vi "LM3Sxxxx_PWM_Config.vi"(8 "error in (no error)":errorcluster, 10 "Config Data":string[](array[string]), 11 "Interrupt Name":string) -> (0 "error out":errorcluster, 3 "Interrupt Configuration":string[](array[string]))   [LabVIEW 2011]
panel:
  in  "PWM 1":string
  in  "PWM 0":string
  in  "Invert output":bool
  in  "Disable on fault":bool
  in  "Invert output":bool
  in  "Disable on fault":bool
  in  "help":bool
  in  "Duty cycle units":u32(ring) items=["Percent", "Hundredths percent", "PWM duty cycle"]
  in  "Duty cycle units":u32(ring) items=["Percent", "Hundredths percent", "PWM duty cycle"]
  in  "Duty cycle":u32=50
  in  "Duty cycle":u32=50
  in  "Enable":bool
  in  "Enable":bool=TRUE
  in  "Zero":bool
  in  "Compare B":bool
  in  "Compare A":bool
  in  "Load":bool
  in  "Center alignment":bool
  in  "Frequency (Hz)":u32=1000
  in  "cancel":bool
  in  "ok":bool
  in  "PWM divider":u32(ring) items=["/1", "/2", "/4", "/8", "/16", "/32", "/64"]
  # "Interrupts"
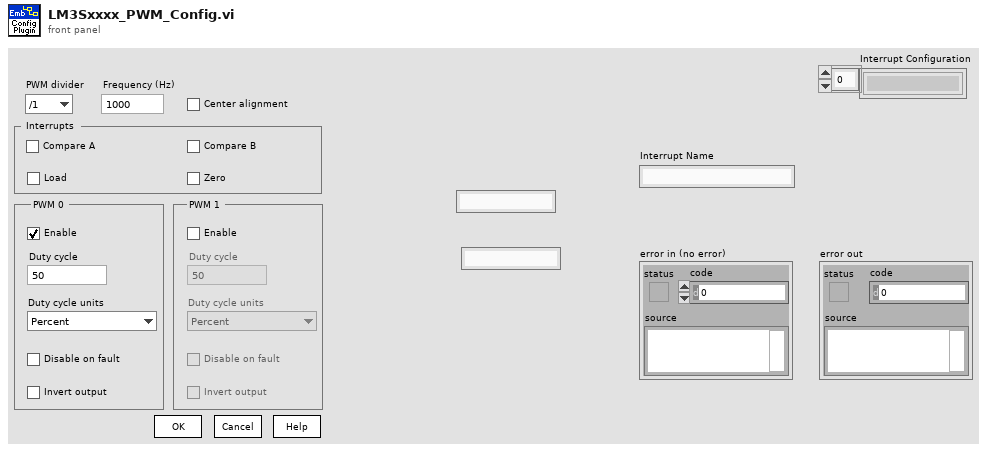
[diagram p1: front panel]
types:
  T1 = enum8{"Enabled", "Disabled", "Disabled and Grayed Out"}
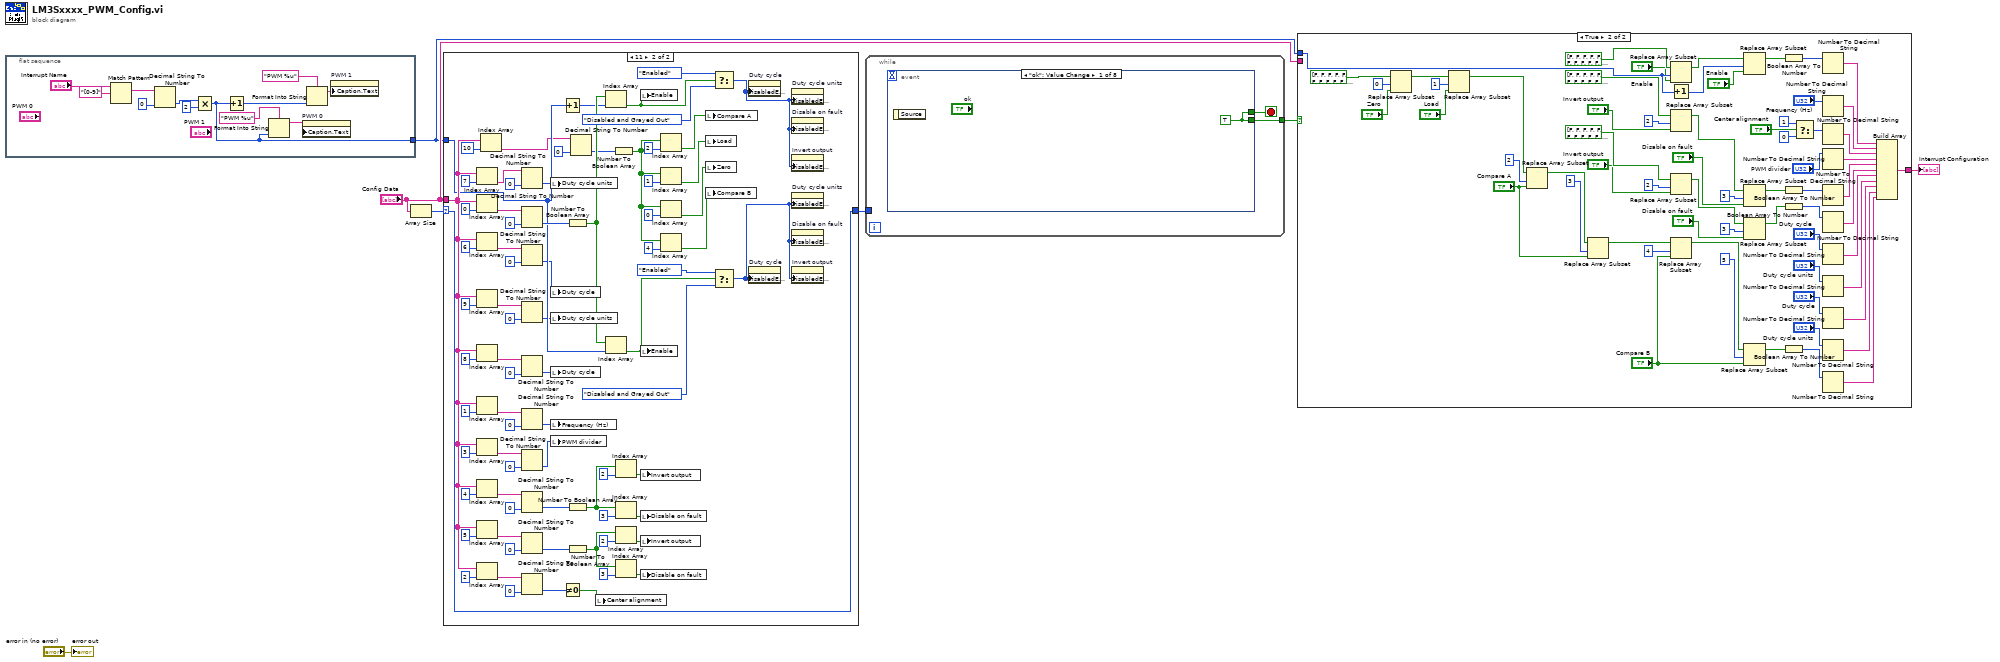
[diagram p0: block diagram]
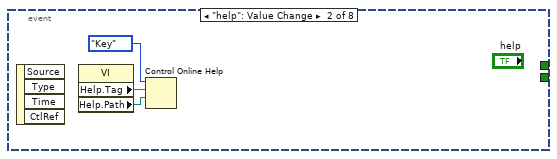
[diagram p4: hidden frame]
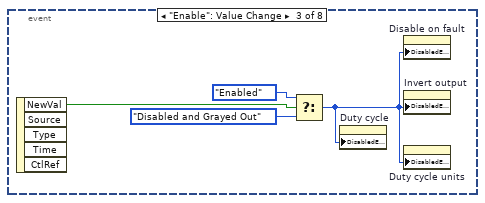
[diagram p5: hidden frame]
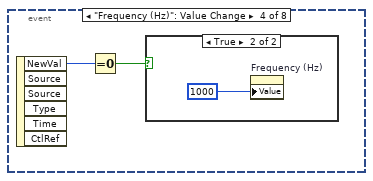
[diagram p6: hidden frame]
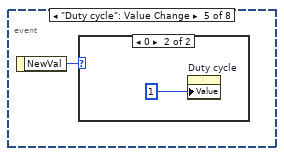
[diagram p8: hidden frame]
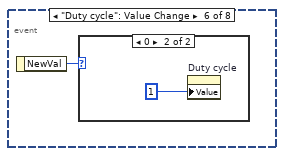
[diagram p10: hidden frame]
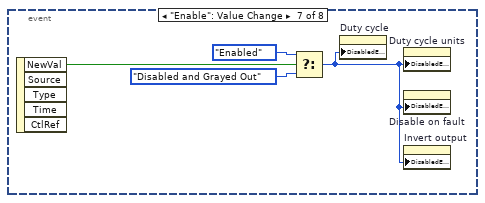
[diagram p12: hidden frame]
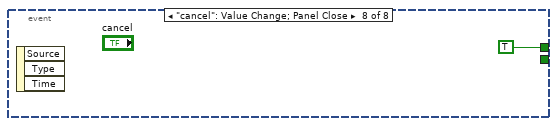
[diagram p13: hidden frame]
diagram:
  n1 = flat-sequence {
    tunnel: [w10] -> w1
    frame #0 {
      n2 = Match Pattern(string="Interrupt Name", regular expression="[0-9]") -> (match substring=w16:string)  [unwired: 1 in, 3 out]
      n3 = Decimal String To Number(string=w16, default (0L)=u32 0) -> (number=w9:u32)  [unwired: 1 in, 1 out]
      n4 = Multiply(x=w9, y=2) -> (x*y=w10:u32)
      n5 = Increment(x=w10) -> (x+1=w12:u32)
      n6 = Format Into String(format string="PWM %u", w10) -> (resulting string=w14:string)  [unwired: 2 in, 1 out]
      n7 = property on="PWM 0" class="Str"("Caption.Text"=w14) -> ()  [unwired: 2 in, 2 out]
      n8 = Format Into String(format string="PWM %u", w12) -> (resulting string=w11:string)  [unwired: 2 in, 1 out]
      n9 = property on="PWM 1" class="Str"("Caption.Text"=w11) -> ()  [unwired: 2 in, 2 out]
    }
  }
  n10 = Array Size(array="Config Data") -> (size(s)=w4:i32)
  n11 = case shown="11" w4 {
    selector: w4 -> [w20 w85]
    tunnel: "Config Data" -> [_ w86]
    tunnel: [w20 w85] -> w2
    tunnel: w1 -> [_ w80]
    frame Default {
    }
    frame 11 {
      n12 = Index Array(array=w86, index=7) -> (element=w25:string)
      n13 = Index Array(array=w86, index=0) -> (element=w84:string)
      n14 = Index Array(array=w86, index=6) -> (element=w43:string)
      n15 = Index Array(array=w86, index=9) -> (element=w22:string)
      n16 = Index Array(array=w86, index=8) -> (element=w40:string)
      n17 = Index Array(array=w86, index=1) -> (element=w70:string)
      n18 = Index Array(array=w86, index=3) -> (element=w64:string)
      n19 = Index Array(array=w86, index=4) -> (element=w59:string)
      n20 = Index Array(array=w86, index=5) -> (element=w58:string)
      n21 = Index Array(array=w86, index=2) -> (element=w68:string)
      n22 = Index Array(array=w86, index=10) -> (element=w36:string)
      n23 = Decimal String To Number(string=w25, default (0L)=u32 0) -> (number=w24:u32)  [unwired: 1 in, 1 out]
      n24 = Decimal String To Number(string=w84, default (0L)=u32 0) -> (number=w83:u32)  [unwired: 1 in, 1 out]
      n25 = Decimal String To Number(string=w43, default (0L)=u32 0) -> (number=w42:u32)  [unwired: 1 in, 1 out]
      n26 = Decimal String To Number(string=w22, default (0L)=u32 0) -> (number=w21:u32)  [unwired: 1 in, 1 out]
      n27 = Decimal String To Number(string=w40, default (0L)=u32 0) -> (number=w39:u32)  [unwired: 1 in, 1 out]
      n28 = Decimal String To Number(string=w70, default (0L)=u32 0) -> (number=w69:u32)  [unwired: 1 in, 1 out]
      n29 = Decimal String To Number(string=w64, default (0L)=u32 0) -> (number=w63:u32)  [unwired: 1 in, 1 out]
      n30 = Decimal String To Number(string=w59, default (0L)=u32 0) -> (number=w57:u32)  [unwired: 1 in, 1 out]
      n31 = Decimal String To Number(string=w58, default (0L)=u32 0) -> (number=w56:u32)  [unwired: 1 in, 1 out]
      n32 = Decimal String To Number(string=w68, default (0L)=u32 0) -> (number=w66:u32)  [unwired: 1 in, 1 out]
      n33 = local write "Duty cycle units"(w24) -> ()
      n34 = local write "Duty cycle"(w42) -> ()
      n35 = local write "Duty cycle units"(w21) -> ()
      n36 = local write "Duty cycle"(w39) -> ()
      n37 = local write "Frequency (Hz)"(w69) -> ()
      n38 = local write "PWM divider"(w63) -> ()
      n39 = Increment(x=w80) -> (x+1=w79:u32)
      n40 = Not Equal To 0?(x=w66) -> (x != 0?=w65:bool)
      n41 = Number To Boolean Array(number=w83) -> (Boolean array=w81:bool[])
      n42 = Number To Boolean Array(number=w57) -> (Boolean array=w54:bool[])
      n43 = Number To Boolean Array(number=w56) -> (Boolean array=w53:bool[])
      n44 = Decimal String To Number(string=w36, default (0L)=u32 0) -> (number=w37:u32)  [unwired: 1 in, 1 out]
      n45 = local write "Center alignment"(w65) -> ()
      n46 = Index Array(array=w81, index=w79) -> (element=w72:bool)
      n47 = Index Array(array=w81, index=w80) -> (element=w76:bool)
      n48 = Number To Boolean Array(number=w37) -> (Boolean array=w35:bool[])
      n49 = Index Array(array=w54, index=2) -> (element=w48:bool)
      n50 = Index Array(array=w54, index=3) -> (element=w45:bool)
      n51 = Index Array(array=w53, index=2) -> (element=w47:bool)
      n52 = Index Array(array=w53, index=3) -> (element=w46:bool)
      n53 = local write "Enable"(w72) -> ()
      n54 = local write "Enable"(w76) -> ()
      n55 = local write "Invert output"(w48) -> ()
      n56 = local write "Disable on fault"(w45) -> ()
      n57 = local write "Invert output"(w47) -> ()
      n58 = local write "Disable on fault"(w46) -> ()
      n59 = Index Array(array=w35, index=2) -> (element=w32:bool)
      n60 = Index Array(array=w35, index=1) -> (element=w31:bool)
      n61 = Index Array(array=w35, index=0) -> (element=w34:bool)
      n62 = Index Array(array=w35, index=4) -> (element=w33:bool)
      n63 = local write "Compare A"(w32) -> ()
      n64 = local write "Load"(w31) -> ()
      n65 = local write "Zero"(w34) -> ()
      n66 = local write "Compare B"(w33) -> ()
      n67 = Select(t=T1."Enabled" ("Disabled"), s=w72, f=T1."Disabled and Grayed Out" ("Disabled")) -> (s? t:f=w75:T1)
      n68 = Select(t=T1."Enabled" ("Disabled"), s=w76, f=T1."Disabled and Grayed Out" ("Disabled")) -> (s? t:f=w78:T1)
      n69 = property on="Duty cycle" class="DigNum (strict)"("DisabledEnum"=w75) -> ()  [unwired: 2 in, 2 out]
      n70 = property on="Duty cycle" class="DigNum (strict)"("DisabledEnum"=w78) -> ()  [unwired: 2 in, 2 out]
      n71 = property on="Duty cycle units" class="Ring (strict)"("DisabledEnum"=w75) -> ()  [unwired: 2 in, 2 out]
      n72 = property on="Disable on fault" class="Bool (strict)"("DisabledEnum"=w75) -> ()  [unwired: 2 in, 2 out]
      n73 = property on="Invert output" class="Bool (strict)"("DisabledEnum"=w75) -> ()  [unwired: 2 in, 2 out]
      n74 = property on="Duty cycle units" class="Ring (strict)"("DisabledEnum"=w78) -> ()  [unwired: 2 in, 2 out]
      n75 = property on="Disable on fault" class="Bool (strict)"("DisabledEnum"=w78) -> ()  [unwired: 2 in, 2 out]
      n76 = property on="Invert output" class="Bool (strict)"("DisabledEnum"=w78) -> ()  [unwired: 2 in, 2 out]
    }
  }
  n77 = while {
    tunnel: [w98] -> w6
    tunnel: w2 -> [_]
    stop <- w99 stop-if-true
    n78 = event shown="[0] \"ok\": Value Change" {
      selector: _ -> [_ _ _ _ _ _ _ _]
      dyn-events: _ -> [_ _ _ _ _ _ _ _]
      timeout: _ -> [_ _ _ _ _ _ _ _]
      tunnel: [w100 _ _ _ _ _ _ TRUE] -> w99
      tunnel: [w100 _ _ _ _ _ _ _] -> w98
      event "ok": Value Change {
        w100 = TRUE
        n79 = event-data() -> ()  [unwired: 2 out]
      }
      event "help": Value Change {
        n80 = event-data() -> ()  [unwired: 5 out]
        n81 = property class="VI"() -> ("Help.Tag"=w101:string, "Help.Path"=w102:path)  [unwired: 2 in, 2 out]
        n82 = Control Online Help(2:w102, 3:w101, 4:enum16{"Contents", "Key", "Close"}."Key" ("Operation")) -> ()  [unwired: 1 in, 1 out]
      }
      event "Enable": Value Change {
        n83 = event-data() -> ("NewVal"=w104:bool)  [unwired: 5 out]
        n84 = Select(t=T1."Enabled" ("Disabled"), s=w104, f=T1."Disabled and Grayed Out" ("Disabled")) -> (s? t:f=w105:T1)
        n85 = property on="Duty cycle" class="DigNum (strict)"("DisabledEnum"=w105) -> ()  [unwired: 2 in, 2 out]
        n86 = property on="Disable on fault" class="Bool (strict)"("DisabledEnum"=w105) -> ()  [unwired: 2 in, 2 out]
        n87 = property on="Invert output" class="Bool (strict)"("DisabledEnum"=w105) -> ()  [unwired: 2 in, 2 out]
        n88 = property on="Duty cycle units" class="Ring (strict)"("DisabledEnum"=w105) -> ()  [unwired: 2 in, 2 out]
      }
      event "Frequency (Hz)": Value Change {
        n89 = event-data() -> ("NewVal"=w109:u32)  [unwired: 6 out]
        n90 = Equal To 0?(x=w109) -> (x = 0?=w108:bool)
        n91 = case shown="True" w108 {
          frame False {
          }
          frame True {
            n92 = property on="Frequency (Hz)" class="DigNum (strict)"("Value"=u32 1000 ("Frequency (Hz)")) -> ()  [unwired: 2 in, 2 out]
          }
        }
      }
      event "Duty cycle": Value Change {
        n93 = event-data() -> ("NewVal"=w111:u32)  [unwired: 1 out]
        n94 = case shown="0" w111 {
          frame Default {
          }
          frame 0 {
            n95 = property on="Duty cycle" class="DigNum (strict)"("Value"=u32 1 ("Duty cycle")) -> ()  [unwired: 2 in, 2 out]
          }
        }
      }
      event "Duty cycle": Value Change {
        n96 = event-data() -> ("NewVal"=w113:u32)  [unwired: 1 out]
        n97 = case shown="0" w113 {
          frame Default {
          }
          frame 0 {
            n98 = property on="Duty cycle" class="DigNum (strict)"("Value"=u32 1 ("Duty cycle")) -> ()  [unwired: 2 in, 2 out]
          }
        }
      }
      event "Enable": Value Change {
        n99 = event-data() -> ("NewVal"=w115:bool)  [unwired: 5 out]
        n100 = Select(t=T1."Enabled" ("Disabled"), s=w115, f=T1."Disabled and Grayed Out" ("Disabled")) -> (s? t:f=w116:T1)
        n101 = property on="Duty cycle" class="DigNum (strict)"("DisabledEnum"=w116) -> ()  [unwired: 2 in, 2 out]
        n102 = property on="Duty cycle units" class="Ring (strict)"("DisabledEnum"=w116) -> ()  [unwired: 2 in, 2 out]
        n103 = property on="Disable on fault" class="Bool (strict)"("DisabledEnum"=w116) -> ()  [unwired: 2 in, 2 out]
        n104 = property on="Invert output" class="Bool (strict)"("DisabledEnum"=w116) -> ()  [unwired: 2 in, 2 out]
      }
      event "cancel": Value Change; Panel Close {
        n105 = event-data() -> ()  [unwired: 4 out]
      }
    }
  }
  n106 = case shown="True" w6 {
    tunnel: "Config Data" -> [w120 _]
    tunnel: [w120 w184] -> w5
    tunnel: w1 -> [_ w143]
    frame False {
    }
    frame True {
      n107 = Replace Array Subset(array=bool[] [FALSE, FALSE, FALSE, FALSE, FALSE, FALSE, FALSE, FALSE, FALSE, FALSE, FALSE, FALSE, FALSE, FALSE, FALSE, FALSE, FALSE, FALSE, FALSE, FALSE, FALSE, FALSE, FALSE, FALSE, FALSE, FALSE, FALSE, FALSE, FALSE, FALSE, FALSE, FALSE], new element="Zero", index=0) -> (w138:bool[])
      n108 = Replace Array Subset(array=w138, new element="Load", index=1) -> (w137:bool[])
      n109 = Replace Array Subset(array=w137, new element="Compare A", index=2) -> (w136:bool[])
      n110 = Replace Array Subset(array=w136, new element="Compare A", index=3) -> (w133:bool[])
      n111 = Replace Array Subset(array=bool[] [FALSE, FALSE, FALSE, FALSE, FALSE, FALSE, FALSE, FALSE, FALSE, FALSE, FALSE, FALSE, FALSE, FALSE, FALSE, FALSE, FALSE, FALSE, FALSE, FALSE, FALSE, FALSE, FALSE, FALSE, FALSE, FALSE, FALSE, FALSE, FALSE, FALSE, FALSE, FALSE], new element="Enable", index=w143) -> (w147:bool[])
      n112 = Increment(x=w143) -> (x+1=w142:u32)
      n113 = Replace Array Subset(array=bool[] [FALSE, FALSE, FALSE, FALSE, FALSE, FALSE, FALSE, FALSE, FALSE, FALSE, FALSE, FALSE, FALSE, FALSE, FALSE, FALSE, FALSE, FALSE, FALSE, FALSE, FALSE, FALSE, FALSE, FALSE, FALSE, FALSE, FALSE, FALSE, FALSE, FALSE, FALSE, FALSE], new element="Invert output", index=2) -> (w173:bool[])
      n114 = Replace Array Subset(array=bool[] [FALSE, FALSE, FALSE, FALSE, FALSE, FALSE, FALSE, FALSE, FALSE, FALSE, FALSE, FALSE, FALSE, FALSE, FALSE, FALSE, FALSE, FALSE, FALSE, FALSE, FALSE, FALSE, FALSE, FALSE, FALSE, FALSE, FALSE, FALSE, FALSE, FALSE, FALSE, FALSE], new element="Invert output", index=2) -> (w163:bool[])
      n115 = Replace Array Subset(array=w133, new element="Compare B", index=4) -> (w132:bool[])
      n116 = Replace Array Subset(array=w147, new element="Enable", index=w142) -> (w146:bool[])
      n117 = Replace Array Subset(array=w173, new element="Disable on fault", index=3) -> (w171:bool[])
      n118 = Replace Array Subset(array=w163, new element="Disable on fault", index=3) -> (w162:bool[])
      n119 = Replace Array Subset(array=w132, new element="Compare B", index=5) -> (w131:bool[])
      n120 = Boolean Array To Number(Boolean array=w146) -> (number=w145:u32)
      n121 = Boolean Array To Number(Boolean array=w171) -> (number=w170:u32)
      n122 = Boolean Array To Number(Boolean array=w162) -> (number=w161:u32)
      n123 = Boolean Array To Number(Boolean array=w131) -> (number=w135:u32)
      n124 = Select(t=u32 1, s="Center alignment", f=u32 0) -> (s? t:f=w178:u32)
      n125 = Number To Decimal String(number=w145) -> (decimal integer string=w144:string)  [unwired: 1 in]
      n126 = Number To Decimal String(number="Frequency (Hz)") -> (decimal integer string=w182:string)  [unwired: 1 in]
      n127 = Number To Decimal String(number=w178) -> (decimal integer string=w177:string)  [unwired: 1 in]
      n128 = Number To Decimal String(number="PWM divider") -> (decimal integer string=w175:string)  [unwired: 1 in]
      n129 = Number To Decimal String(number=w170) -> (decimal integer string=w172:string)  [unwired: 1 in]
      n130 = Number To Decimal String(number=w161) -> (decimal integer string=w165:string)  [unwired: 1 in]
      n131 = Number To Decimal String(number="Duty cycle") -> (decimal integer string=w155:string)  [unwired: 1 in]
      n132 = Number To Decimal String(number="Duty cycle units") -> (decimal integer string=w153:string)  [unwired: 1 in]
      n133 = Number To Decimal String(number="Duty cycle") -> (decimal integer string=w151:string)  [unwired: 1 in]
      n134 = Number To Decimal String(number="Duty cycle units") -> (decimal integer string=w149:string)  [unwired: 1 in]
      n135 = Number To Decimal String(number=w135) -> (decimal integer string=w134:string)  [unwired: 1 in]
      n136 = Build Array(w144, w182, w177, w175, w172, w165, w155, w153, w151, w149, w134) -> (w184:string[])
    }
  }
  "Interrupt Configuration" <- w5
  "error out" <- "error in (no error)"
